vi "Initialize Client Proxy LNA.vi"(8 "error in (no error)":errorcluster, 10 "Network Actor in":refnum<class "Client Proxy LNA.lvclass">, 11 "Server Controller in":refnum<class "Server Controller.lvclass">) -> (0 "error out":errorcluster, 2 "Caller-To-Actor Enqueuer":refnum<class "Message Enqueuer.lvclass">, 3 "Server Controller out":refnum<class "Server Controller.lvclass">)   [LabVIEW 2016, in "Server Controller.lvlib" / "Server Controller.lvclass"]
uses:
  Server Controller.lvclass
  C:/Program Files (x86)/National Instruments/LabVIEW 2016/vi.lib/ActorFramework/Actor/Actor.lvclass
  <vilib>/ActorFramework/Message Enqueuer/Message Enqueuer.lvclass
  Client Proxy LNA/Client Proxy LNA.lvclass
  <vilib>/ActorFramework/Actor/Actor.lvclass/Actor.ctl
  <vilib>/ActorFramework/Message Enqueuer/Message Enqueuer.lvclass/Message Enqueuer.ctl
  <vilib>/ActorFramework/Message Enqueuer/Init from Existing Queue.vi
  <vilib>/ActorFramework/Actor/Actor.lvclass
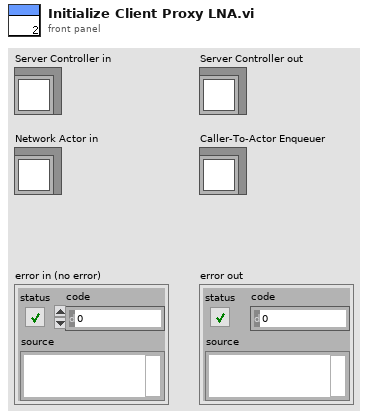
[diagram p1: front panel]
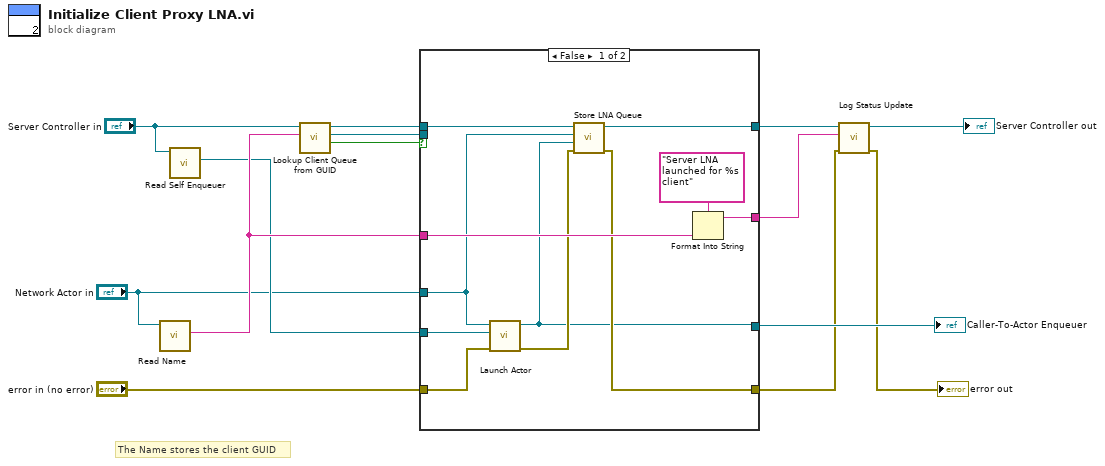
[diagram p0: block diagram]
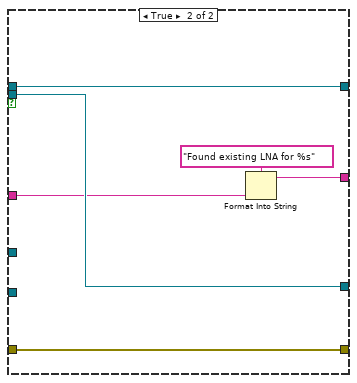
[diagram p2: hidden frame]
diagram:
  # "The Name stores the client GUID"
  n1 = call-dynamic "Read Name.vi"("Network Actor in"="Network Actor in") -> ("Name"=w14:string)  [unwired: 10 in]
  n2 = call <vilib>:"Read Self Enqueuer.vi"("Actor"="Server Controller in") -> ("Self Enqueuer"=w8:refnum<class "Message Enqueuer.lvclass">)  [unwired: 10 in]
  n3 = call "Lookup Client Queue from GUID.vi"("GUID"=w14, "Server Controller in"="Server Controller in") -> ("found"=w11:bool, "Caller-To-Actor Enqueuer"=w12:refnum<class "Message Enqueuer.lvclass">, "Server Controller out"=w13:refnum<class "Server Controller.lvclass">)  [unwired: 6 in, 1 out]
  n4 = case shown="False" w11 {
    tunnel: "error in (no error)" -> [w25 w30]
    tunnel: w8 -> [w24 _]
    tunnel: "Network Actor in" -> [w16 _]
    tunnel: [w15 w31] -> w9
    tunnel: [w17 w30] -> w3
    tunnel: w12 -> [_ w31]
    tunnel: w13 -> [w23 w29]
    tunnel: [w22 w29] -> w6
    tunnel: w14 -> [w20 w27]
    tunnel: [w19 w28] -> w5
    frame False {
      n5 = call <vilib>:"Launch Actor.vi"("error in (no error)"=w25, "Actor-to-Caller Enqueuer"=w24, "Actor"=w16) -> ("error out"=w18:errorcluster, "Caller-To-Actor Enqueuer"=w15:refnum<class "Message Enqueuer.lvclass">)  [unwired: 7 in]
      n6 = call "Store LNA Queue.vi"("error in (no error)"=w18, "Message Enqueuer in"=w15, "Network Actor in"=w16, "Server Controller in"=w23) -> ("error out"=w17:errorcluster, "Server Controller out"=w22:refnum<class "Server Controller.lvclass">)  [unwired: 6 in]
      n7 = Format Into String(format string="Server LNA launched for %s client" ("String"), w20) -> (resulting string=w19:string)  [unwired: 2 in, 1 out]
    }
    frame True {
      n8 = Format Into String(format string="Found existing LNA for %s", w27) -> (resulting string=w28:string)  [unwired: 2 in, 1 out]
    }
  }
  "Caller-To-Actor Enqueuer" <- w9
  n9 = call-dynamic "Log Status Update.vi"("error in (no error)"=w3, "String"=w5, "Controller in"=w6) -> ("error out"=→"error out":errorcluster, "Controller out"=→"Server Controller out":refnum<class "Server Controller.lvclass">)  [unwired: 7 in]
